vi "array page up.vi"(8 "error in (no error)":errorcluster, 11 "Array in":refnum<vi>) -> (0 "error out":errorcluster)   [LabVIEW 2014, in "Tagbus PID Module editor node.lvclass"]
uses:
  Tagbus PID Module editor node.lvclass
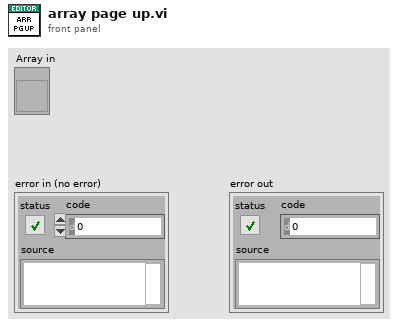
[diagram p1: front panel]
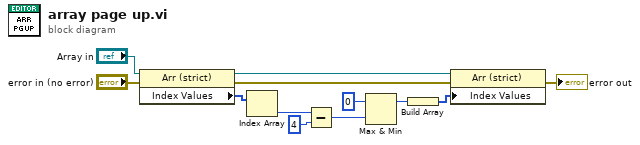
[diagram p0: block diagram]
diagram:
  n1 = property class="Arr (strict)"(reference="Array in", error in="error in (no error)") -> (reference out=w4:refnum<vi>, error out=w1:errorcluster, "Index Values"=w6:u32[])
  n2 = Index Array(array=w6) -> (element=w7:u32)  [unwired: 1 in]
  n3 = Subtract(x=w7, y=u32 4) -> (x-y=w9:u32)
  n4 = Max & Min(x=u32 0, y=w9) -> (max(x,y)=w11:u32)  [unwired: 1 out]
  n5 = Build Array(w11) -> (w10:u32[])
  n6 = property class="Arr (strict)"(reference=w4, error in=w1, "Index Values"=w10) -> (error out=→"error out":errorcluster)  [unwired: 1 out]
